vi "Loop_SM.vi"() -> ()   [LabVIEW 2017, in "Gimbal.lvlib"]
uses:
  Gimbal.lvlib
  ENUM_SM_State.ctl
  TypeDef/Cluster_Gimbal CMD.ctl
  TypeDef/Cluster_Gimbal Axis CMD.ctl
  TypeDef/ENUM_Gimbal CMD Mode.ctl
  ENUM_SM_Action.ctl
  Globals/Global_STOP.vi
  Global_CMD.vi
  Global_SM Write_Data Out.vi
panel:
  out "LeftRightAngle":i32
  out "UpDownAngle":i32
  out "Cycle Time (S)":dbl format="%.3g"
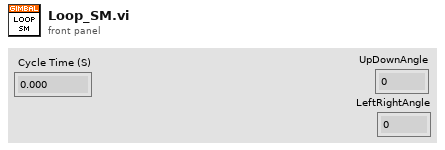
[diagram p1: front panel]
types:
  T1 = typedef "Cluster_Gimbal CMD.ctl" = cluster{"UpDown":T2, "LeftRight":T2}
  T2 = typedef "Cluster_Gimbal Axis CMD.ctl" = cluster{"Cmd":T3, "Value":dbl}
  T3 = typedef "ENUM_Gimbal CMD Mode.ctl" = enum16{"Angle", "Error"}
  T4 = typedef "Gimbal.lvlib/ENUM_SM_State.ctl" = enum16{"Startup", "Idle", "Shutdown"}
  T5 = typedef "Gimbal.lvlib/ENUM_SM_Action.ctl" = enum16{"No Action", "Reset Time", "Reset All", "Action A", "Action B"}
  T6 = cluster{"State":T4, "Previous State":T4, "Current Time":timestamp, "Previous Time":timestamp, "Start Time":timestamp, "Target Time (ms)":u32, "Cycle Time(S)":dbl, "UpDownAngle":i32, "LeftRightAngle":i32, "SM OutputI INT":i32, "SM Output Bool":bool, "CMD_Gimbal":T1}
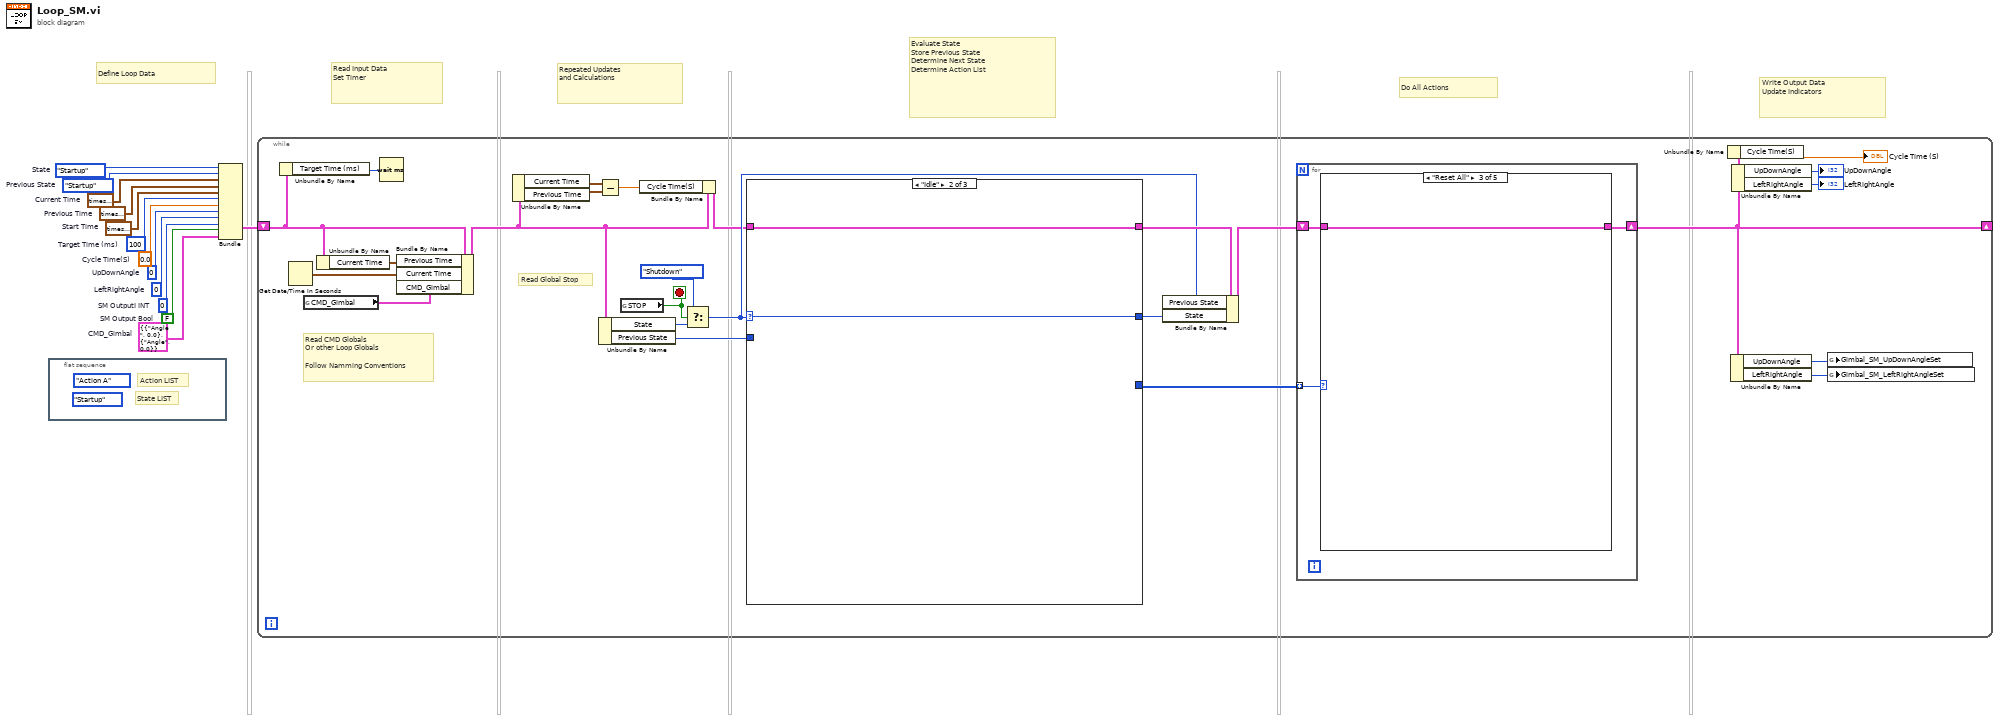
[diagram p0: block diagram]
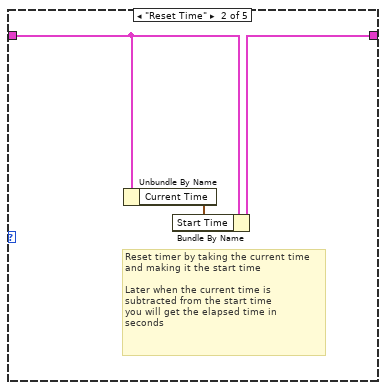
[diagram p3: hidden frame]
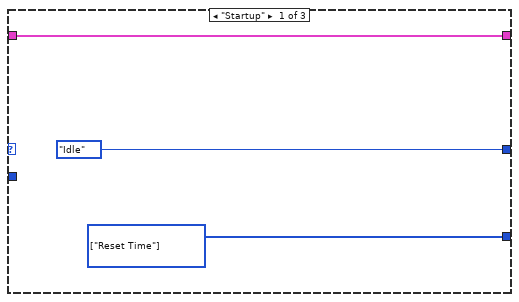
[diagram p6: hidden frame]
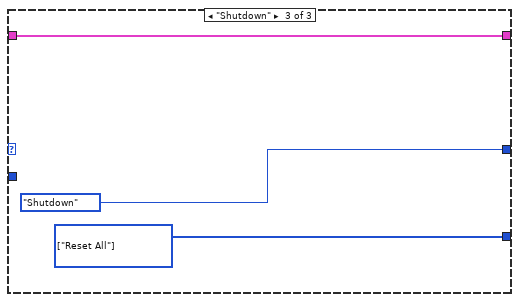
[diagram p7: hidden frame]
diagram:
  w1 = T1 {"UpDown"={"Cmd"=enum."Angle", "Value"=0.0}, "LeftRight"={"Cmd"=enum."Angle", "Value"=0.0}}  # CMD_Gimbal
  w2 = 0  # LeftRightAngle
  w3 = 0  # UpDownAngle
  w4 = 0.0  # Cycle Time(S)
  w5 = ENUM_SM_State."Startup"  # Previous State
  w6 = timestamp(0 s since 1904-01-01)  # Previous Time
  w7 = FALSE  # SM Output Bool
  w8 = 0  # SM OutputI INT
  w9 = u32 100  # Target Time (ms)
  w10 = timestamp(0 s since 1904-01-01)  # Start Time
  w11 = timestamp(0 s since 1904-01-01)  # Current Time
  w12 = ENUM_SM_State."Startup"  # State
  # "Define Loop Data"
  # "Repeated Updates\nand Calculations"
  # "Read Input Data\nSet Timer"
  # "Evaluate State\nStore Previous State\nDetermine Next State\nDetermine Action List"
  # "Do All Actions"
  # "Write Output Data\nUpdate Indicators"
  n1 = flat-sequence {
    frame #0 {
      (unwired) ENUM_SM_State."Startup" ("State")
      (unwired) ENUM_SM_Action."Action A" ("Action")
      # "State LIST"
      # "Action LIST"
    }
  }
  n2 = Bundle("State"=w12, "Previous State"=w5, "Current Time"=w11, "Previous Time"=w6, "Start Time"=w10, "Target Time (ms)"=w9, "Cycle Time(S)"=w4, "UpDownAngle"=w3, "LeftRightAngle"=w2, "SM OutputI INT"=w8, "SM Output Bool"=w7, "CMD_Gimbal"=w1) -> (w13:T6)  [unwired: 1 in]
  n3 = while {
    shift-right: [w26] -> _
    shift-left: w13 -> [w29]
    stop <- w34 stop-if-true
    # "Read CMD Globals\nOr other Loop Globals\n\nFollow Namming Conventions"
    # "Read Global Stop"
    n4 = Unbundle By Name(w29) -> ("Target Time (ms)"=w31:u32)
    n5 = Get Date/Time In Seconds() -> (seconds since 1Jan1904=w38:timestamp)
    n6 = global read "Global_CMD.vi" "CMD_Gimbal"() -> (w18:T1)
    n7 = Unbundle By Name(w29) -> ("Current Time"=w30:timestamp)
    n8 = Wait (ms)(milliseconds to wait=w31) -> ()  [unwired: 1 out]
    n9 = Bundle By Name(cluster=w29, "Previous Time"=w30, "Current Time"=w38, "CMD_Gimbal"=w18) -> (w22:T6)
    n10 = Unbundle By Name(w22) -> ("Current Time"=w23:timestamp, "Previous Time"=w24:timestamp)
    n11 = Subtract(x=w23, y=w24) -> (x-y=w20:dbl)
    n12 = Unbundle By Name(w22) -> ("State"=w32:T4, "Previous State"=w28:T4)
    n13 = global read "Global_STOP.vi" "STOP"() -> (w34:bool)
    n14 = Bundle By Name(cluster=w22, "Cycle Time(S)"=w20) -> (w21:T6)
    n15 = Select(t=ENUM_SM_State."Shutdown" ("State"), s=w34, f=w32) -> (s? t:f=w27:T4)
    n16 = case shown="\"Idle\"" w27 {
      selector: w27 -> [_ w52 _]
      tunnel: w21 -> [w51 w53 w56]
      tunnel: [w51 w53 w56] -> w36
      tunnel: [ENUM_SM_State."Idle" ("State") w52 ENUM_SM_State."Shutdown" ("State")] -> w35
      tunnel: [w50 _ w54] -> w19
      tunnel: w28 -> [_ _ _]
      frame "Startup" {
        w50 = T5[] [enum."Reset Time"] items=["No Action", "Reset Time", "Reset All", "Action A", "Action B"] ("Actions")
      }
      frame "Idle" {
      }
      frame "Shutdown" {
        w54 = T5[] [enum."Reset All"] items=["No Action", "Reset Time", "Reset All", "Action A", "Action B"] ("Actions")
      }
    }
    n17 = Bundle By Name(cluster=w36, "Previous State"=w27, "State"=w35) -> (w37:T6)
    n18 = for {
      tunnel: w19 -> [w41] mode=indexing
      shift-right: [w40] -> w26
      shift-left: w37 -> [w39]
      n19 = case shown="\"Reset All\"" w41 {
        tunnel: w39 -> [w42 w45 w46 w47 w48]
        tunnel: [w42 w44 w46 w47 w48] -> w40
        frame "No Action" {
        }
        frame "Reset Time" {
          # "Reset timer by taking the current time\nand making it the start time\n\nLater when the current time is \nsubtracted from the start time\nyou will get the elapsed time in \nseconds"
          n20 = Unbundle By Name(w45) -> ("Current Time"=w43:timestamp)
          n21 = Bundle By Name(cluster=w45, "Start Time"=w43) -> (w44:T6)
        }
        frame "Reset All" {
        }
        frame "Action A" {
        }
        frame "Action B" {
        }
      }
    }
    n22 = Unbundle By Name(w26) -> ("Cycle Time(S)"=→"Cycle Time (S)":dbl)
    n23 = Unbundle By Name(w26) -> ("UpDownAngle"=w17:i32, "LeftRightAngle"=w16:i32)
    n24 = Unbundle By Name(w26) -> ("UpDownAngle"=→"UpDownAngle":i32, "LeftRightAngle"=→"LeftRightAngle":i32)
    n25 = global write "Global_SM Write_Data Out.vi" "Gimbal_SM_UpDownAngleSet"(w17) -> ()
    n26 = global write "Global_SM Write_Data Out.vi" "Gimbal_SM_LeftRightAngleSet"(w16) -> ()
  }
